vi "Unconstrained Exponential Fit.vi"(0 "Y":dbl[](array[numeric]), 5 "X":dbl[](array[numeric]), 7 "Weight":dbl[](array[numeric]), 9 "tolerance":dbl=0.0001 format="%#_3g", 11 "method":T1 items=["Least Square", "Least Absolute Residual", "Bisquare"], 12 "refine?":bool) -> (4 "Best Exponential Fit":dbl[](array[numeric]), 6 "amplitude":dbl, 8 "damping":dbl, 14 "residue":dbl, 15 "error":i32)   [LabVIEW 2017, in "NI_AALPro.lvlib"]
doc: "LabVIEW does not support the Unconstrained Exponential Fit VI. Use the Exponential Fit VI instead."
uses:
  <vilib>/Analysis/NI_AALPro.lvlib
  <vilib>/Analysis/6fits.llb/Curve Fitting Criteria.ctl
panel:
  # "Exponential Fit"
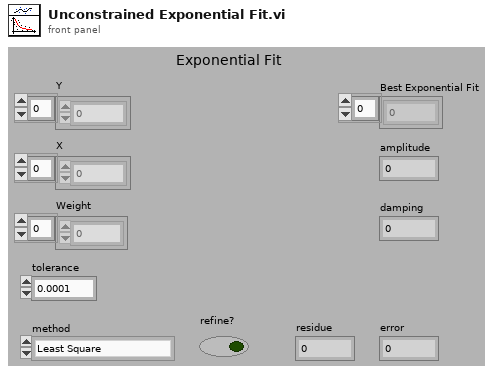
[diagram p1: front panel]
types:
  T1 = typedef "NI_AALPro.lvlib/Curve Fitting Criteria.ctl" = u16
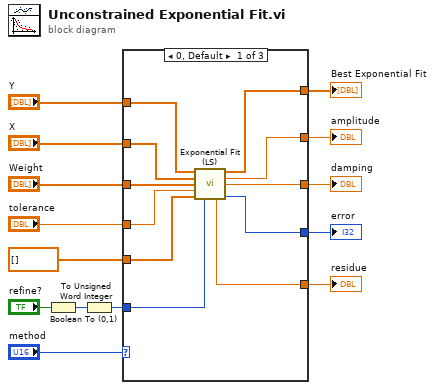
[diagram p0: block diagram]
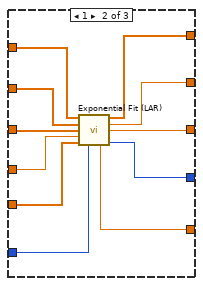
[diagram p2: hidden frame]
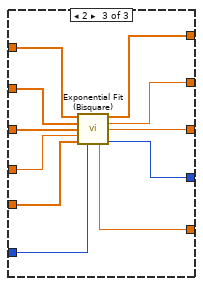
[diagram p3: hidden frame]
diagram:
  n1 = Boolean To (0,1)(Boolean="refine?") -> (0, 1=w2:i16)
  n2 = To Unsigned Word Integer(number=w2) -> (unsigned 16bit integer=w1:u16)
  n3 = case shown="0, Default" "method" {
    tunnel: "Y" -> [w25 w36 w47]
    tunnel: "X" -> [w24 w35 w46]
    tunnel: "Weight" -> [w23 w34 w45]
    tunnel: "tolerance" -> [w22 w33 w44]
    tunnel: dbl[] [] -> [w21 w32 w43]
    tunnel: [w20 w26 w42] -> w10
    tunnel: [w19 w27 w41] -> w9
    tunnel: [w18 w28 w40] -> w8
    tunnel: [w17 w29 w39] -> w6
    tunnel: w1 -> [w16 w31 w37]
    tunnel: [w15 w30 w38] -> w5
    frame 0, Default {
      n4 = call <vilib>:"Exponential Fit (LS).vi"("Y"=w25, "X"=w24, "Weight"=w23, "tolerance"=w22, "Initial Coefficients"=w21, "algorithm"=w16) -> ("Best Exponential Fit"=w20:dbl[], "amplitude"=w19:dbl, "damping"=w18:dbl, "residue"=w15:dbl, "error"=w17:i32)  [unwired: 5 out]
    }
    frame 1 {
      n5 = call <vilib>:"Exponential Fit (LAR).vi"("Y"=w36, "X"=w35, "Weight"=w34, "tolerance"=w33, "Initial Coefficients"=w32, "algorithm"=w31) -> ("Best Exponential Fit"=w26:dbl[], "amplitude"=w27:dbl, "damping"=w28:dbl, "residue"=w30:dbl, "error"=w29:i32)  [unwired: 5 out]
    }
    frame 2 {
      n6 = call <vilib>:"Exponential Fit (Bisquare).vi"("Y"=w47, "X"=w46, "Weight"=w45, "tolerance"=w44, "Initial Coefficients"=w43, "algorithm"=w37) -> ("Best Exponential Fit"=w42:dbl[], "amplitude"=w41:dbl, "damping"=w40:dbl, "residue"=w38:dbl, "error"=w39:i32)  [unwired: 5 out]
    }
  }
  "error" <- w6
  "amplitude" <- w9
  "damping" <- w8
  "Best Exponential Fit" <- w10
  "residue" <- w5
